vi "探头启用设置.vi"() -> ()   [LabVIEW 2022 SP3, in "斯坦道多参数.lvlib"]
uses:
  <vilib>/Utility/miscctls.llb/LVPointTypeDef.ctl
panel:
  in  "余氯启用":bool
  in  "SS":bool
  in  "悬浮物探头选择":T1
  in  "水中油启用":bool
  in  "氨氮启用":bool
  in  "氯化物启用":bool
  in  "藻密度单位":enum16{"cells/mL", "cells/L"}(ring)
  in  "叶绿素a单位":enum16{"μg/L", "mg/L"}(ring)
  in  "关闭":bool
  in  "水温通道":u16(ring)=1 items=["pH", "DO", "浊度", "电导率", "叶绿素a", "藻密度"]
  in  "DO2探头选择":T1=enum."国弘"
  in  "DO2启用":bool
  in  "COD探头选择":T1=enum."国弘"
  in  "COD启用":bool
  in  "pH":bool
  in  "DO":bool
  in  "Turb":bool
  in  "Cond":bool
  in  "Temp":bool
  in  "叶绿素a启用":bool
  in  "藻密度":bool
  in  "pH探头选择":T1
  in  "DO探头选择":T1
  in  "电导率探头选择":T1
  in  "浊度探头选择":T1
  in  "叶绿素a探头选择":T1
  in  "藻密度探头选择":T1
  in  "ORP启用":bool
  in  "ORP探头选择":T1
  # "请选择要启用的参数"
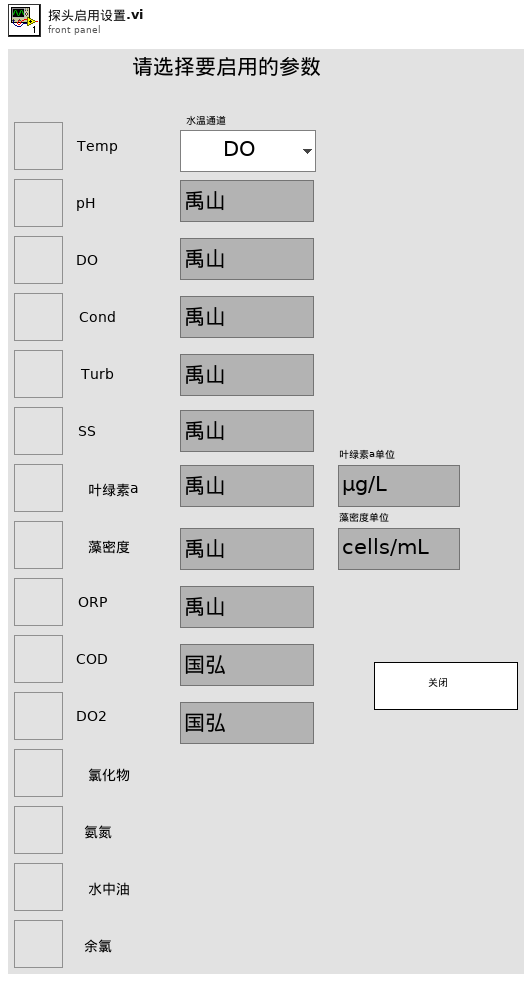
[diagram p1: front panel]
types:
  T1 = typedef "斯坦道多参数.lvlib/探头类型.ctl" = enum16{"禹山", "国弘", "纳清", "STD"}
  T2 = typedef "LVPointTypeDef.ctl" = cluster{"Horizontal":i16, "Vertical":i16}
  T3 = cluster{"pH探头选择":T1, "DO探头选择":T1, "电导率探头选择":T1, "浊度探头选择":T1, "悬浮物探头选择":T1, "叶绿素a探头选择":T1, "蓝绿藻探头选择":T1, "orp探头选择":T1, "COD探头选择":T1, "DO2探头选择":T1, "氨氮探头选择":T1, "水中油探头选择":T1, "余氯探头选择":T1}
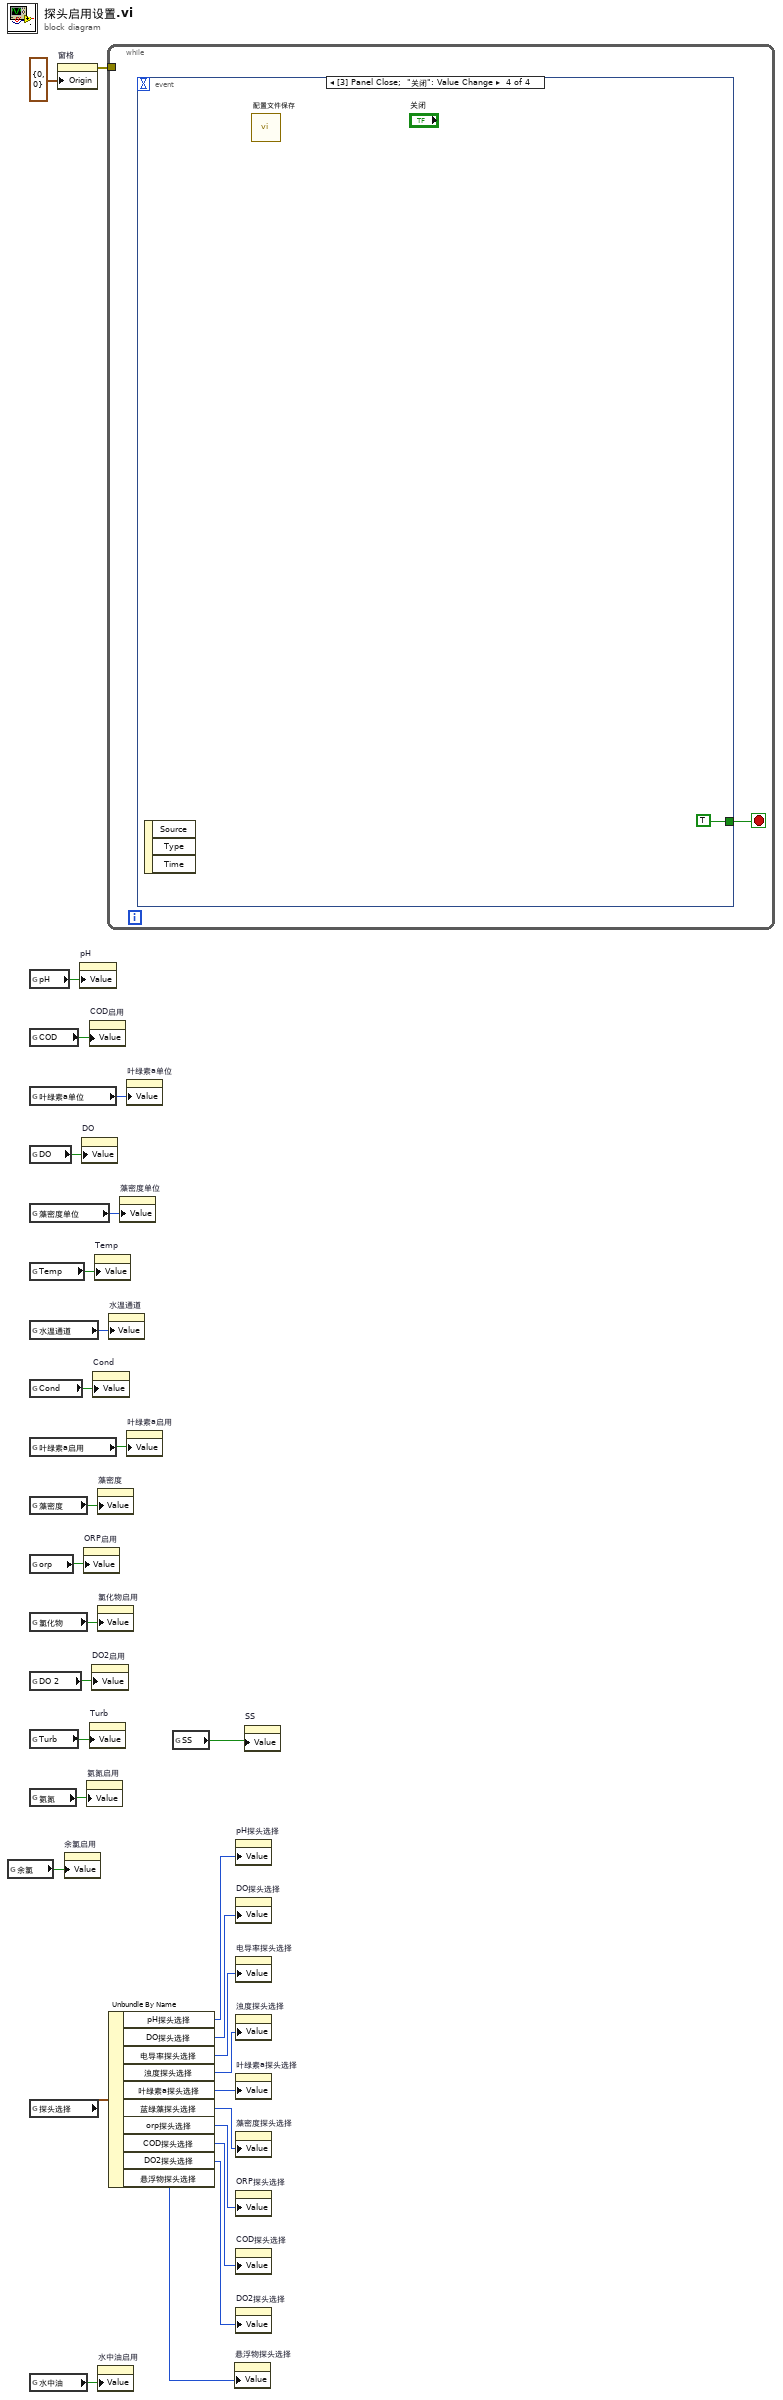
[diagram p0: block diagram]
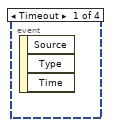
[diagram p2: hidden frame]
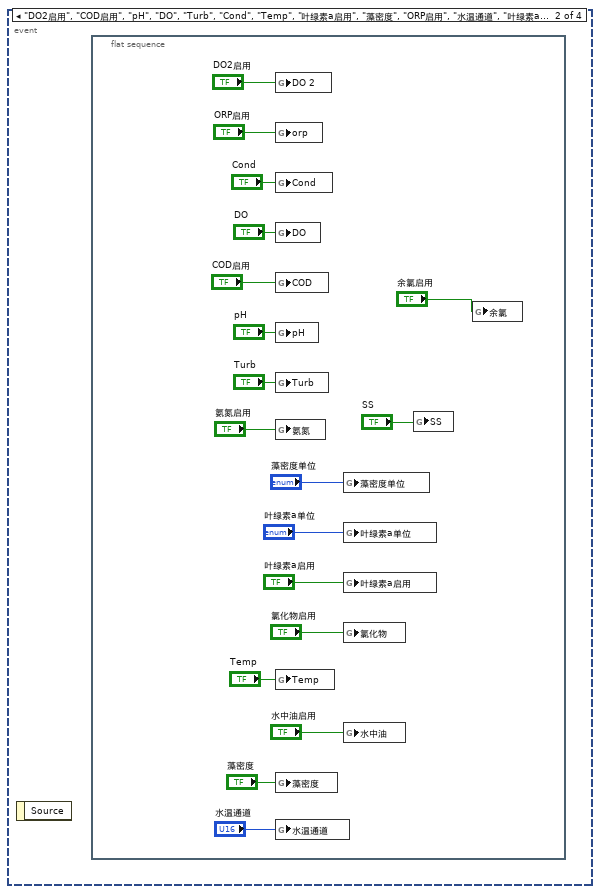
[diagram p3: hidden frame]
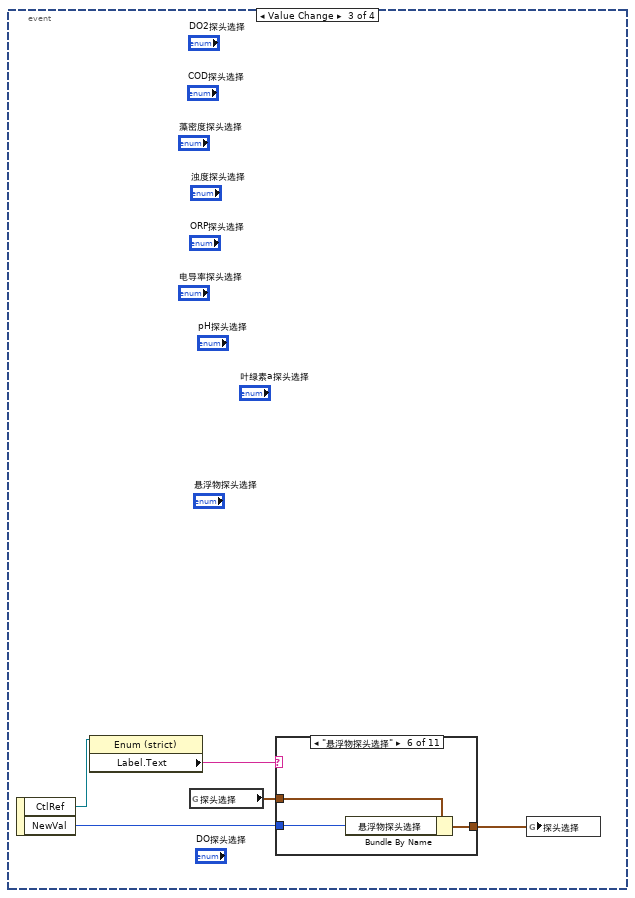
[diagram p4: hidden frame]
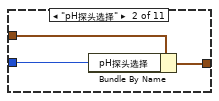
[diagram p6: hidden frame]
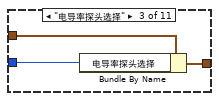
[diagram p7: hidden frame]
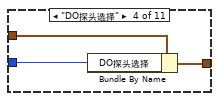
[diagram p8: hidden frame]
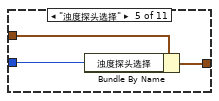
[diagram p9: hidden frame]
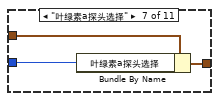
[diagram p10: hidden frame]
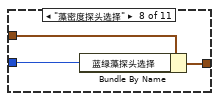
[diagram p11: hidden frame]
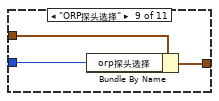
[diagram p12: hidden frame]
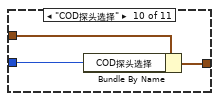
[diagram p13: hidden frame]
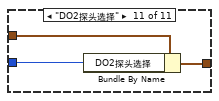
[diagram p14: hidden frame]
diagram:
  n1 = global read "断电保存变量.vi" "余氯"() -> (w1:bool)
  n2 = global read "断电保存变量.vi" "pH"() -> (w29:bool)
  n3 = global read "断电保存变量.vi" "COD"() -> (w28:bool)
  n4 = global read "断电保存变量.vi" "叶绿素a单位"() -> (w8:enum16{"μg/L", "mg/L"})
  n5 = global read "断电保存变量.vi" "DO"() -> (w27:bool)
  n6 = global read "断电保存变量.vi" "藻密度单位"() -> (w9:enum16{"cells/mL", "cells/L"})
  n7 = global read "断电保存变量.vi" "Temp"() -> (w26:bool)
  n8 = global read "断电保存变量.vi" "水温通道"() -> (w25:enum16{"pH", "DO", "浊度", "电导率", "叶绿素a", "藻密度"})
  n9 = global read "断电保存变量.vi" "Cond"() -> (w24:bool)
  n10 = global read "断电保存变量.vi" "叶绿素a启用"() -> (w23:bool)
  n11 = global read "断电保存变量.vi" "藻密度"() -> (w22:bool)
  n12 = global read "断电保存变量.vi" "orp"() -> (w21:bool)
  n13 = global read "断电保存变量.vi" "氯化物"() -> (w7:bool)
  n14 = global read "断电保存变量.vi" "DO 2"() -> (w20:bool)
  n15 = global read "断电保存变量.vi" "Turb"() -> (w19:bool)
  n16 = global read "断电保存变量.vi" "氨氮"() -> (w6:bool)
  n17 = global read "断电保存变量.vi" "探头选择"() -> (w18:T3)
  n18 = global read "断电保存变量.vi" "水中油"() -> (w5:bool)
  n19 = property on="窗格" class="Pane"("Origin"=T2 {"Horizontal"=0, "Vertical"=0} ("原点")) -> (error out=w30:errorcluster)  [unwired: 2 in, 1 out]
  n20 = property on="余氯启用" class="Bool (strict)"("Value"=w1) -> ()  [unwired: 2 in, 2 out]
  n21 = property on="pH" class="Bool (strict)"("Value"=w29) -> ()  [unwired: 2 in, 2 out]
  n22 = property on="DO" class="Bool (strict)"("Value"=w27) -> ()  [unwired: 2 in, 2 out]
  n23 = property on="ORP启用" class="Bool (strict)"("Value"=w21) -> ()  [unwired: 2 in, 2 out]
  n24 = property on="氨氮启用" class="Bool (strict)"("Value"=w6) -> ()  [unwired: 2 in, 2 out]
  n25 = property on="COD启用" class="Bool (strict)"("Value"=w28) -> ()  [unwired: 2 in, 2 out]
  n26 = property on="Turb" class="Bool (strict)"("Value"=w19) -> ()  [unwired: 2 in, 2 out]
  n27 = property on="DO2启用" class="Bool (strict)"("Value"=w20) -> ()  [unwired: 2 in, 2 out]
  n28 = property on="Cond" class="Bool (strict)"("Value"=w24) -> ()  [unwired: 2 in, 2 out]
  n29 = property on="Temp" class="Bool (strict)"("Value"=w26) -> ()  [unwired: 2 in, 2 out]
  n30 = property on="藻密度" class="Bool (strict)"("Value"=w22) -> ()  [unwired: 2 in, 2 out]
  n31 = property on="氯化物启用" class="Bool (strict)"("Value"=w7) -> ()  [unwired: 2 in, 2 out]
  n32 = property on="水中油启用" class="Bool (strict)"("Value"=w5) -> ()  [unwired: 2 in, 2 out]
  n33 = while {
    tunnel: w30 -> [_]
    stop <- w32 stop-if-true
    n34 = event shown="[3] Panel Close;  \"关闭\": Value Change" {
      selector: _ -> [_ _ _ _]
      dyn-events: _ -> [_ _ _ _]
      timeout: _ -> [_ _ _ _]
      tunnel: [_ _ _ TRUE] -> w32
      event Timeout {
        n35 = event-data() -> ()  [unwired: 1 in, 3 out]
      }
      event "DO2启用", "COD启用", "pH", "DO", "Turb", "Cond", "Temp", "叶绿素a启用", "藻密度", "ORP启用", "水温通道", "叶绿素a单位", "藻密度单位", "氯化物启用", "氨氮启用", "水中油启用", "SS", "余氯启用": Value Change {
        n36 = event-data() -> ()  [unwired: 1 in, 1 out]
        n37 = flat-sequence {
          frame #0 {
            n38 = global write "断电保存变量.vi" "DO 2"("DO2启用") -> ()
            n39 = global write "断电保存变量.vi" "orp"("ORP启用") -> ()
            n40 = global write "断电保存变量.vi" "Cond"("Cond") -> ()
            n41 = global write "断电保存变量.vi" "DO"("DO") -> ()
            n42 = global write "断电保存变量.vi" "COD"("COD启用") -> ()
            n43 = global write "断电保存变量.vi" "pH"("pH") -> ()
            n44 = global write "断电保存变量.vi" "Turb"("Turb") -> ()
            n45 = global write "断电保存变量.vi" "氨氮"("氨氮启用") -> ()
            n46 = global write "断电保存变量.vi" "Temp"("Temp") -> ()
            n47 = global write "断电保存变量.vi" "藻密度"("藻密度") -> ()
            n48 = global write "断电保存变量.vi" "水温通道"("水温通道") -> ()
            n49 = global write "断电保存变量.vi" "藻密度单位"("藻密度单位") -> ()
            n50 = global write "断电保存变量.vi" "叶绿素a单位"("叶绿素a单位") -> ()
            n51 = global write "断电保存变量.vi" "叶绿素a启用"("叶绿素a启用") -> ()
            n52 = global write "断电保存变量.vi" "氯化物"("氯化物启用") -> ()
            n53 = global write "断电保存变量.vi" "水中油"("水中油启用") -> ()
            n54 = global write "断电保存变量.vi" "SS"("SS") -> ()
            n55 = global write "断电保存变量.vi" "余氯"("余氯启用") -> ()
          }
        }
      }
      event Value Change {
        n56 = event-data() -> ("CtlRef"=w52:refnum<vi>, "NewVal"=w51:T1)  [unwired: 1 in]
        n57 = property class="Enum (strict)"(reference=w52) -> ("Label.Text"=w55:string)  [unwired: 1 in, 2 out]
        n58 = global read "断电保存变量.vi" "探头选择"() -> (w54:T3)
        n59 = case shown="\"悬浮物探头选择\"" w55 {
          tunnel: w54 -> [w56 w59 w62 w65 w68 w71 w74 w77 w80 w83 w86]
          tunnel: [w56 w58 w61 w64 w67 w70 w73 w76 w79 w82 w85] -> w53
          tunnel: w51 -> [_ w57 w60 w63 w66 w69 w72 w75 w78 w81 w84]
          frame Default {
          }
          frame "pH探头选择" {
            n60 = Bundle By Name(cluster=w59, "pH探头选择"=w57) -> (w58:T3)
          }
          frame "电导率探头选择" {
            n61 = Bundle By Name(cluster=w62, "电导率探头选择"=w60) -> (w61:T3)
          }
          frame "DO探头选择" {
            n62 = Bundle By Name(cluster=w65, "DO探头选择"=w63) -> (w64:T3)
          }
          frame "浊度探头选择" {
            n63 = Bundle By Name(cluster=w68, "浊度探头选择"=w66) -> (w67:T3)
          }
          frame "悬浮物探头选择" {
            n64 = Bundle By Name(cluster=w71, "悬浮物探头选择"=w69) -> (w70:T3)
          }
          frame "叶绿素a探头选择" {
            n65 = Bundle By Name(cluster=w74, "叶绿素a探头选择"=w72) -> (w73:T3)
          }
          frame "藻密度探头选择" {
            n66 = Bundle By Name(cluster=w77, "蓝绿藻探头选择"=w75) -> (w76:T3)
          }
          frame "ORP探头选择" {
            n67 = Bundle By Name(cluster=w80, "orp探头选择"=w78) -> (w79:T3)
          }
          frame "COD探头选择" {
            n68 = Bundle By Name(cluster=w83, "COD探头选择"=w81) -> (w82:T3)
          }
          frame "DO2探头选择" {
            n69 = Bundle By Name(cluster=w86, "DO2探头选择"=w84) -> (w85:T3)
          }
        }
        n70 = global write "断电保存变量.vi" "探头选择"(w53) -> ()
      }
      event Panel Close; "关闭": Value Change {
        n71 = event-data() -> ()  [unwired: 1 in, 3 out]
        n72 = call "配置文件保存.vi"() -> ()  [unwired: 12 in]
      }
    }
  }
  n73 = property on="水温通道" class="Ring (strict)"("Value"=w25) -> ()  [unwired: 2 in, 2 out]
  n74 = Unbundle By Name(w18) -> ("pH探头选择"=w4:T1, "DO探头选择"=w17:T1, "电导率探头选择"=w16:T1, "浊度探头选择"=w15:T1, "叶绿素a探头选择"=w14:T1, "蓝绿藻探头选择"=w13:T1, "orp探头选择"=w12:T1, "COD探头选择"=w11:T1, "DO2探头选择"=w10:T1, "悬浮物探头选择"=w2:T1)
  n75 = property on="藻密度单位" class="Enum (strict)"("Value"=w9) -> ()  [unwired: 2 in, 2 out]
  n76 = property on="叶绿素a单位" class="Enum (strict)"("Value"=w8) -> ()  [unwired: 2 in, 2 out]
  n77 = property on="叶绿素a启用" class="Bool (strict)"("Value"=w23) -> ()  [unwired: 2 in, 2 out]
  n78 = global read "断电保存变量.vi" "SS"() -> (w3:bool)
  n79 = property on="悬浮物探头选择" class="Enum (strict)"("Value"=w2) -> ()  [unwired: 2 in, 2 out]
  n80 = property on="pH探头选择" class="Enum (strict)"("Value"=w4) -> ()  [unwired: 2 in, 2 out]
  n81 = property on="DO探头选择" class="Enum (strict)"("Value"=w17) -> ()  [unwired: 2 in, 2 out]
  n82 = property on="电导率探头选择" class="Enum (strict)"("Value"=w16) -> ()  [unwired: 2 in, 2 out]
  n83 = property on="浊度探头选择" class="Enum (strict)"("Value"=w15) -> ()  [unwired: 2 in, 2 out]
  n84 = property on="叶绿素a探头选择" class="Enum (strict)"("Value"=w14) -> ()  [unwired: 2 in, 2 out]
  n85 = property on="藻密度探头选择" class="Enum (strict)"("Value"=w13) -> ()  [unwired: 2 in, 2 out]
  n86 = property on="ORP探头选择" class="Enum (strict)"("Value"=w12) -> ()  [unwired: 2 in, 2 out]
  n87 = property on="COD探头选择" class="Enum (strict)"("Value"=w11) -> ()  [unwired: 2 in, 2 out]
  n88 = property on="DO2探头选择" class="Enum (strict)"("Value"=w10) -> ()  [unwired: 2 in, 2 out]
  n89 = property on="SS" class="Bool (strict)"("Value"=w3) -> ()  [unwired: 2 in, 2 out]
